vi "Reading Group.vi"() -> ()   [LabVIEW 2023]
uses:
  a2659fa0-4576-44a2-ac78-0d942f5ce711.vi
  <userlib>/DAQNavi Polymorphic VI/create/DAQNavi Create Channel(DI-Digital Input).vi
  <userlib>/DAQNavi Polymorphic VI/read/DAQNavi Read (Digital U8 1Chan 1Samp).vi
  <vilib>/addons/TestStand/_TSUtility.llb/TestStand - Set Property Value (Boolean).vi
panel:
  in  "stop":bool
  in  "Sequence Context In":refnum<k7>
  out "error out":errorcluster
  in  "error in":errorcluster
  out "DO group values":bool[](array[boolean])
  out "data":u8
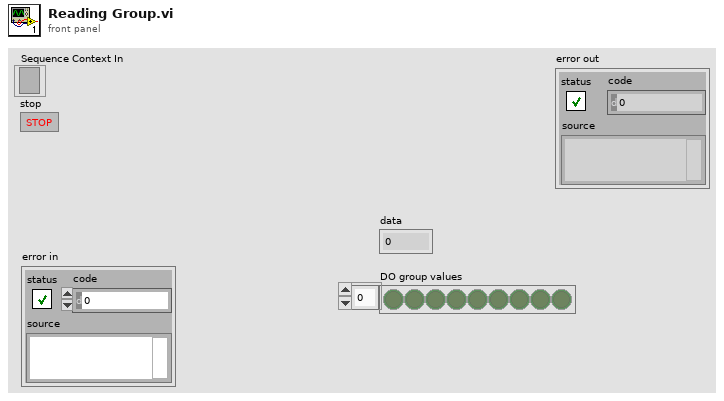
[diagram p1: front panel]
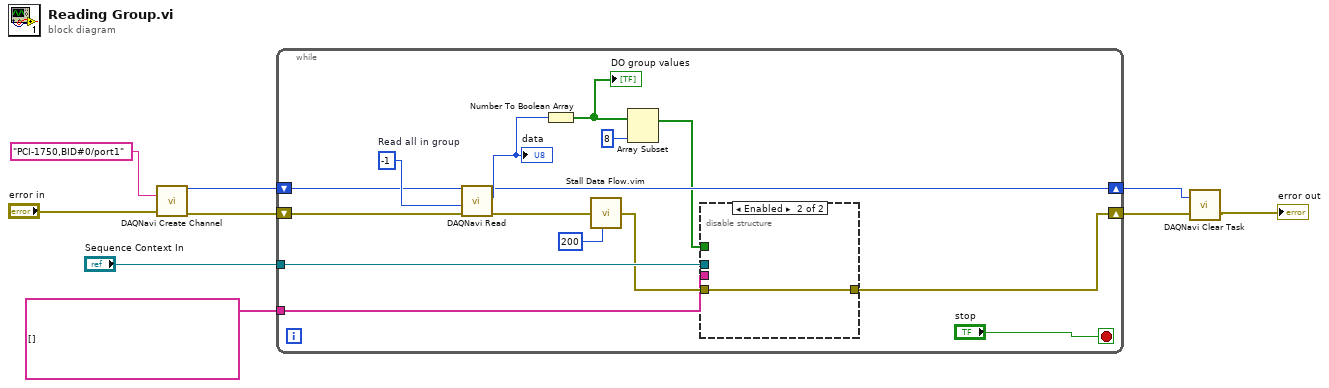
[diagram p0: block diagram]
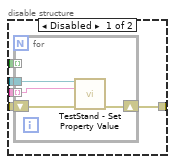
[diagram p2: hidden frame]
diagram:
  n1 = call-poly <userlib>:"DAQNavi Create Channel.vi"("physical channels"="PCI-1750,BID#0/port1" ("Physical channels in"), "error in (no error)"="error in") -> ("task out"=w6:i32, "error out"=w7:errorcluster)  [unwired: 3 in, 9 out]
  n2 = while {
    shift-right: [w15] -> w4
    shift-left: w7 -> [w22]
    shift-right: [w20] -> w5
    shift-left: w6 -> [w21]
    tunnel: "Sequence Context In" -> [w17]
    tunnel: string[] [] ("Lookup String") -> [w11]
    stop <- "stop" stop-if-true
    w24 = -1  # Read all in group
    n3 = call-poly <userlib>:"DAQNavi Read.vi"("error in (no error)"=w22, "portBit"=w24, "task in"=w21) -> ("error out"=w19:errorcluster, "data"=w23:u8, "task out"=w20:i32)  [unwired: 1 in, 5 out]
    "data" <- w23
    n4 = Number To Boolean Array(number=w23) -> (Boolean array=w13:bool[])
    "DO group values" <- w13
    n5 = call "Stall Data Flow.vim"("value in"=w19, "milliseconds to wait"=u32 200) -> ("value out"=w16:errorcluster)  [unwired: 1 out]
    n6 = Array Subset(array=w13, length=8) -> (w14:bool[])  [unwired: 1 in]
    n7 = disable-structure shown="Enabled" {
      disable-tunnel: w17 -> [w29 _]
      disable-tunnel: w16 -> [w28 w34]
      disable-tunnel: [w27 w34] -> w15
      disable-tunnel: w14 -> [w26 _]
      disable-tunnel: w11 -> [w25 _]
      frame Disabled {
        n8 = for {
          tunnel: w29 -> [w33]
          shift-right: [w31] -> w27
          shift-left: w28 -> [w32]
          tunnel: w26 -> [_] mode=indexing
          tunnel: w25 -> [w30] mode=indexing
          n9 = call-poly <vilib>:"TestStand - Set Property Value.vi"("Sequence Context In"=w33, "Lookup String"=w30, "error in (no error)"=w32) -> ("error out"=w31:errorcluster)  [unwired: 11 in, 1 out]
        }
      }
      frame Enabled {
      }
    }
  }
  n10 = call <userlib>:"DAQNavi Clear Task.vi"("error in (no error)"=w4, "task in"=w5) -> ("error out"=→"error out":errorcluster)  [unwired: 1 out]
